vi "INFO.vi"(6 "Message":string, 8 "error in":errorcluster) -> (0 "error out":errorcluster)   [LabVIEW 2020, in "hse-logger.lvlib"]
doc: "Logs a message and the content of the error-cluster.\nAn error on the \"error in\" terminal is duplicated to the \"error dup\" terminal.\n\nDoes not return logging errors!\n\n____\nHAMPEL SOFTWARE ENGINEERING v2.0.6 (2021-04-15 11:38)"
uses:
  hse-logger.lvlib
  Logger/Logger.lvclass
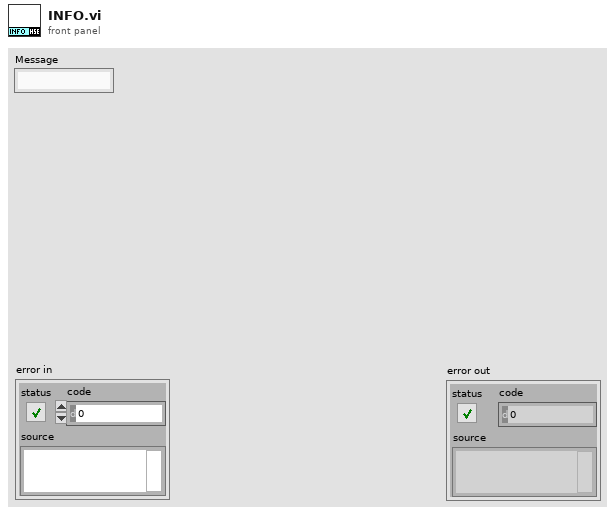
[diagram p1: front panel]
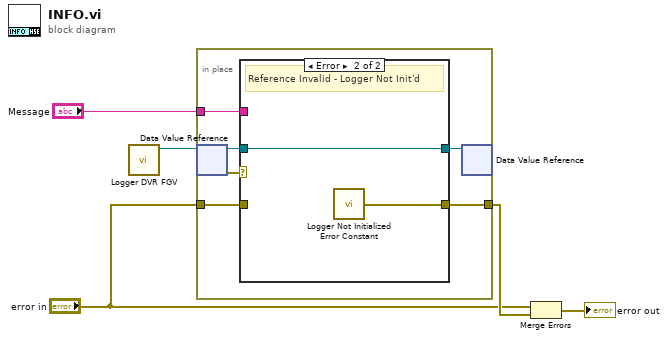
[diagram p0: block diagram]
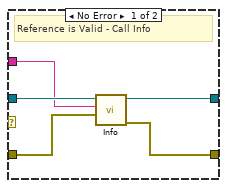
[diagram p2: hidden frame]
diagram:
  n1 = call "Logger DVR FGV.vi"() -> ("Logger DVR"=w3:refnum<data-value>)  [unwired: 10 in, 1 out]
  n2 = in-place {
    in-place-border: "Message" -> [w10]
    in-place-border: [w9] -> w2
    in-place-border: "error in" -> [w6]
    n3 = in-place-dvr #1(w3) -> (w11:refnum<class "Logger.lvclass">, w7:errorcluster)
    n4 = case shown="Error" w7 {
      tunnel: w11 -> [w16 w18]
      tunnel: w10 -> [w15 _]
      tunnel: [w14 w17] -> w9
      tunnel: [w13 w18] -> w8
      tunnel: w6 -> [w12 _]
      frame No Error {
        # "Reference is Valid - Call Info"
        n5 = call-dynamic "Info.vi"("Error to Log"=w12, "Message"=w15, "Logger in"=w16) -> ("error out"=w14:errorcluster, "Logger out"=w13:refnum<class "Logger.lvclass">)  [unwired: 7 in]
      }
      frame Error {
        # "Reference Invalid - Logger Not Init'd"
        n6 = call "Logger Not Initialized Error Constant.vi"() -> ("Logger Not Initialized Error"=w17:errorcluster)
      }
    }
    n7 = in-place-dvr #1(w8) -> ()  [unwired: 2 out]
  }
  n8 = Merge Errors("error in", w2) -> (→"error out":errorcluster)
